vi "Read Outputs.vi"(8 "error in (no error)":errorcluster, 11 "PIOD in":refnum<class "PIOD.lvclass">) -> (0 "error out":errorcluster, 2 "Outputs":bool[](array[boolean]), 3 "PIOD out":refnum<class "PIOD.lvclass">)   [LabVIEW 2018, in "PIOD.lvlib" / "PIOD.lvclass"]
uses:
  PIOD.lvclass
  C:/Users/Ron.Dexter.LUMINARTECH/Desktop/builds/PLC.lvlibp/PLC.lvclass
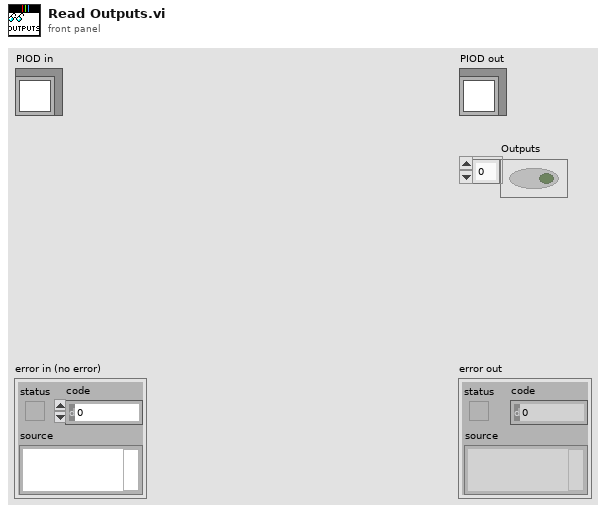
[diagram p1: front panel]
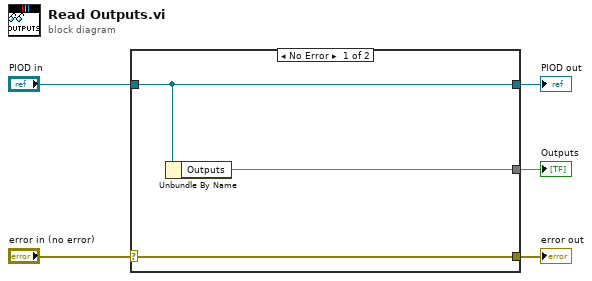
[diagram p0: block diagram]
diagram:
  n1 = case shown="No Error" "error in (no error)" {
    selector: "error in (no error)" -> [w8 w9]
    tunnel: [w8 w9] -> w4
    tunnel: [w7 w10] -> w2
    tunnel: "PIOD in" -> [w7 w10]
    tunnel: [w6 _] -> w1
    frame No Error {
      n2 = Unbundle By Name(w7) -> ("Outputs"=w6)
    }
    frame Error {
    }
  }
  "error out" <- w4
  "PIOD out" <- w2
  "Outputs" <- w1
